vi "Teleop.vi"(10 "Match Info":T2={"Autonomous Elapsed Seconds"=0.0, "TeleOp Elapsed Seconds"=10.261, "Disabled Elapsed Seconds"=2.601, "Visited Autonomous"=FALSE, "Visited TeleOp"=TRUE, "Visited Disabled"=TRUE, "Autonomous Settings"={"Autonomous Style"=enum."Independent", "VI Refnum"=refnum}}, 11 "Call Context":T3=enum."Execute") -> ()   [LabVIEW 2014]
doc: "This VI is called for each TeleOp packet received from the DS where the robot is not disabled. It is often used to read from the joysticks and update I/O or to update setpoints for timed control loops. It should complete and return within 20 milliseconds or it may miss DS packets."
uses:
  <vilib>/Rock Robotics/WPI/DriverStation/WPI_DriverStationDerivedRobotMode.ctl
  <vilib>/Rock Robotics/WPI/DriverStation/WPI_DriverStationMatch Info.ctl
  <vilib>/Rock Robotics/WPI/RobotDrive/WPI_RobotDriveGetSetRefNum.vi
  <vilib>/Rock Robotics/WPI/Joystick/WPI_JoystickGetSetRefNum.vi
  <vilib>/Rock Robotics/Network Tables/SD Write Boolean Array.vi
  <vilib>/Rock Robotics/Network Tables/SD Write Numeric Array.vi
  <vilib>/Rock Robotics/Network Tables/SD Read Boolean.vi
  <vilib>/Rock Robotics/Network Tables/SD Read Number.vi
  <vilib>/Rock Robotics/Network Tables/SD Write Number.vi
  <vilib>/addons/control/pid/pid.llb/PID (DBL).vi
  Robot Global Data.vi
  <vilib>/addons/control/pid/NI_PID_pid.lvlib
panel:
  out "Elevator Rotation Sensor Working":bool
  out "MagneticFieldStrength2 3":u16
  out "MagneticFieldStrength2 2":u16
  out "Diag need to":u8
  out "MagnetFieldStregth":u8
  out "Rotation Sensor Data Out":u8[](array[numeric])
  out "Elevator Power":dbl
  in  "output range":cluster{"output high":dbl, "output low":dbl}={"output high"=0.7, "output low"=-0.7} {"output low" format="%.2f"; "output high" format="%.2f"}
  in  "PID gains":T1={"proportional gain (Kc)"=0.002, "integral time (Ti, min)"=0.0, "derivative time (Td, min)"=0.0} {"derivative time (Td, min)" format="%.3f"; "integral time (Ti, min)" format="%.3f"; "proportional gain (Kc)" format="%.3f"}
  in  "Move Elevator Above Tote Slide":dbl
  out "Claw Encoder Ticks":dbl
  out "Elevator Current":dbl
  out "Claw Current":dbl
  in  "Gain (VoltsPerDegree/Second)":dbl=0.0066
  in  "Reset Zero Position":bool
  out "Angle 3":dbl(knob) scale=0.0..360.0
  out "Angle 2":dbl=-0.0202788065172
  out "Angular Rate 2":dbl=-0.004938670061383929
  out "all currents (A)":dbl[](array[numeric])
  out "Elevator  Encoder Ticks":dbl
  out "Left Encoder Ticks":dbl
  out "Sample Slider 0":dbl(slide) scale=0.0..5.0
  out "Sample Boolean 1":bool
  out "Sample Boolean 0":bool
  # "Right Front"
  # "Right Rear"
  # "Elevator"
  # "Claw"
  # "Right Rear"
  # "Elevator 2"
  # "Left Front"
  # "Left Rear"
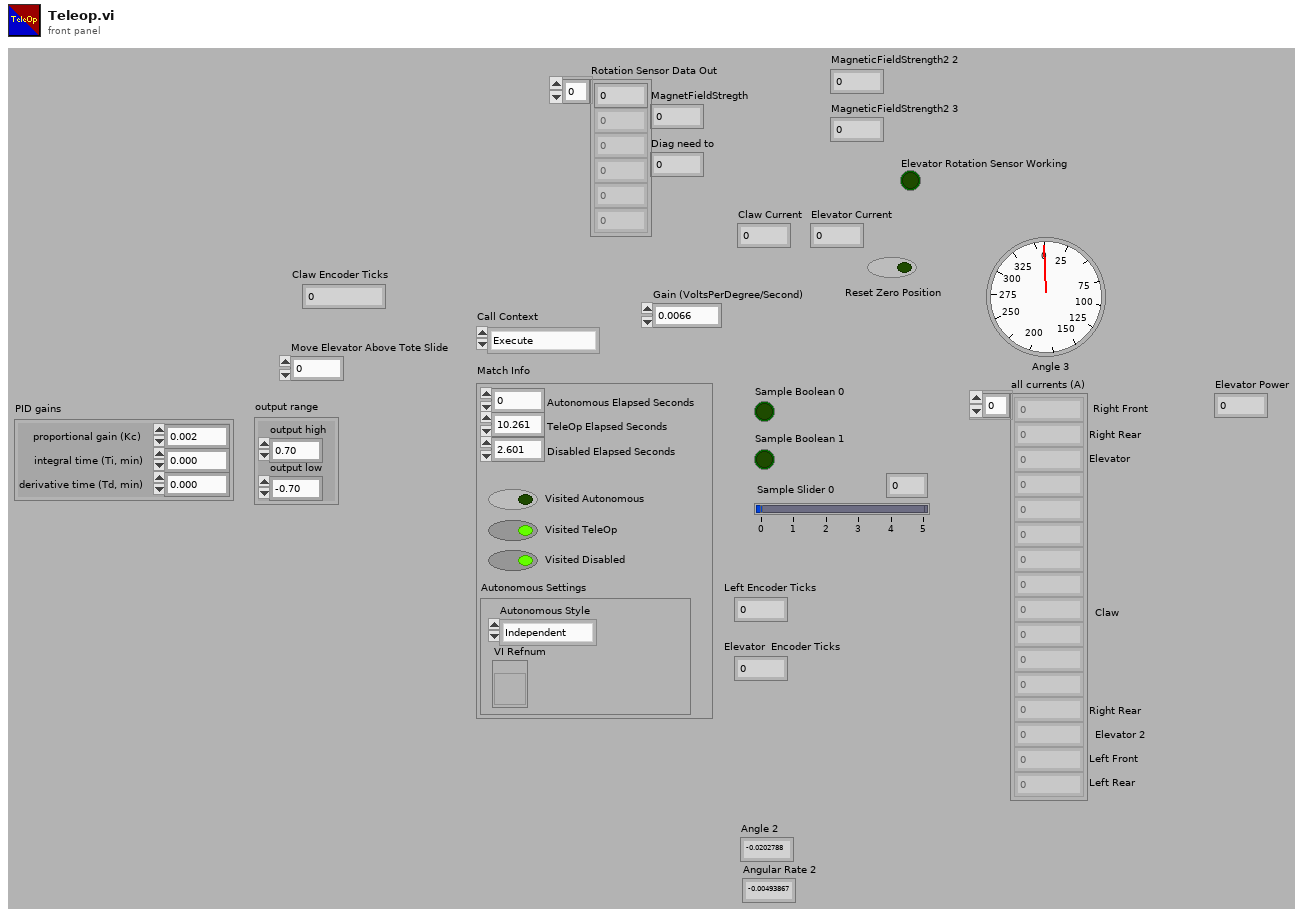
[diagram p1: front panel]
types:
  T1 = cluster{"proportional gain (Kc)":dbl, "integral time (Ti, min)":dbl, "derivative time (Td, min)":dbl}
  T2 = typedef "WPI_DriverStationMatch Info.ctl" = cluster{"Autonomous Elapsed Seconds":dbl, "TeleOp Elapsed Seconds":dbl, "Disabled Elapsed Seconds":dbl, "Visited Autonomous":bool, "Visited TeleOp":bool, "Visited Disabled":bool, "Autonomous Settings":cluster{"Autonomous Style":enum16{"Iterative", "Independent"}, "VI Refnum":refnum<vi>}}
  T3 = typedef "WPI_DriverStationDerivedRobotMode.ctl" = enum16{"Init", "Execute", "Stop"}
  T4 = typedef "WPI_RobotDriveDevRef.ctl" = cluster{"DevStatus":errorcluster, "Motors[]":T5[], "Square Inputs":bool, "Max Output":dbl}
  T5 = typedef "WPI_MotorControlDeviceRef.ctl" = cluster{"DeviceStatus":errorcluster, "Type":T6, "PWM":cluster{"Controller":T7, "PWM Channel":T8, "DeadBand":T9}, "CAN":cluster{"Device Number":u8, "Control Mode":T10, "Semaphore":T11, "Max Vout":dbl, "TalonSRX Control Mode":T12}, "Invert":bool, "TransformRef":T13, "InvTransformRef":T13}
  T6 = typedef "WPI_MotorControlType.ctl" = enum16{"PWM", "CAN", "CANTalonSRX"}
  T7 = typedef "FPGA_TypedefDigitalModule.ctl" = enum16{"Controller 1"}
  T8 = typedef "FPGA_DIOPWMChannel.ctl" = enum8{"PWM 0", "PWM 1", "PWM 2", "PWM 3", "PWM 4", "PWM 5", "PWM 6", "PWM 7", "PWM 8", "PWM 9", "PWM MXP 0", "PWM MXP 1", "PWM MXP 2", "PWM MXP 3", "PWM MXP 4", "PWM MXP 5", "PWM MXP 6", "PWM MXP 7", "PWM MXP 8", "PWM MXP 9", "Invalid"}
  T9 = typedef "WPI_PWMDeadband.ctl" = cluster{"Name":string, "maxPositivePwm":i32, "minPositivePwm":i32, "centerPwm":i32, "maxNegativePwm":i32, "minNegativePwm":i32, "angularRange":u16}
  T10 = typedef "WPI_CANJaguar_ControlMode.ctl" = enum8{"Percent VBus", "Current", "Speed", "Position", "Voltage"}
  T11 = typedef "Semaphore RefNum" = refnum<k1>
  T12 = typedef "WPI_CANTalonSRX_APIControlMode.ctl" = enum8{"Percent VBus", "Speed", "Position", "Slave", "Unchanged / Invalid"}
  T13 = typedef "WPI_PWMTransform_ConPane.ctl" = refnum<vi>
  T14 = typedef "WPI_JoystickDevRef.ctl" = cluster{"Device":T15}
  T15 = typedef "WPI_JoystickDeviceEnum.ctl" = enum16{"USB 0", "USB 1", "USB 2", "USB 3", "USB 4", "USB 5"}
  T16 = typedef "WPI_GyroDevRef.ctl" = cluster{"DevStatus":errorcluster, "Analog Module":T17, "Analog Channel":T18, "Offset":dbl, "Gain (VoltsPerDegree/Second)":dbl}
  T17 = typedef "FPGA_TypedefAnalogModule.ctl" = enum16{"Controller 1"}
  T18 = typedef "FPGA_AIChannel.ctl" = enum8{"AI 0", "AI 1", "AI 2", "AI 3", "AI MXP 0", "AI MXP 1", "AI MXP 2", "AI MXP 3", "Invalid"}
  T19 = typedef "WPI_EncoderDevRef.ctl" = cluster{"DevStatus":errorcluster, "EncoderIndex":T20, "CounterIndex":T21, "DistancePerCount":dbl, "Decoding Type":T22}
  T20 = typedef "FPGA_EncoderIdx.ctl" = enum8{"Enc 0", "Enc 1", "Enc 2", "Enc 3", "Enc 4", "Enc 5", "Enc 6", "Enc 7", "Invalid"}
  T21 = typedef "FPGA_CounterCtrSystemIndex.ctl" = enum8{"Ctr 0", "Ctr 1", "Ctr 2", "Ctr 3", "Ctr 4", "Ctr 5", "Ctr 6", "Ctr 7", "Invalid"}
  T22 = typedef "WPI_EncoderType.ctl" = enum16{"1x", "2x", "4x"}
  T23 = enum16{"Elevator State Bottom", "Elevator State Clear a Tote", "Elevator State Carry a  RC", "Elevator do Nothing"}
  T24 = enum16{"Claw State Open", "Claw State Closed", "Claw State Do Nothing", "Squeeze Hard"}
  T25 = typedef "WPI_I2CDevRef.ctl" = cluster{"DevStatus":errorcluster, "Controller":T7, "Device Address":u8, "Handle":i32, "I2C Bus":T26}
  T26 = typedef "i2c_bus.ctl" = enum16{"I2C On-Board", "I2C MXP", "Invalid"}
  T27 = cluster{"Boolean array[0]":bool, "Boolean array[1]":bool, "Boolean array[2]":bool, "Boolean array[3]":bool, "Boolean array[4]":bool, "Boolean array[5]":bool, "Boolean array[6]":bool, "Boolean array[7]":bool}
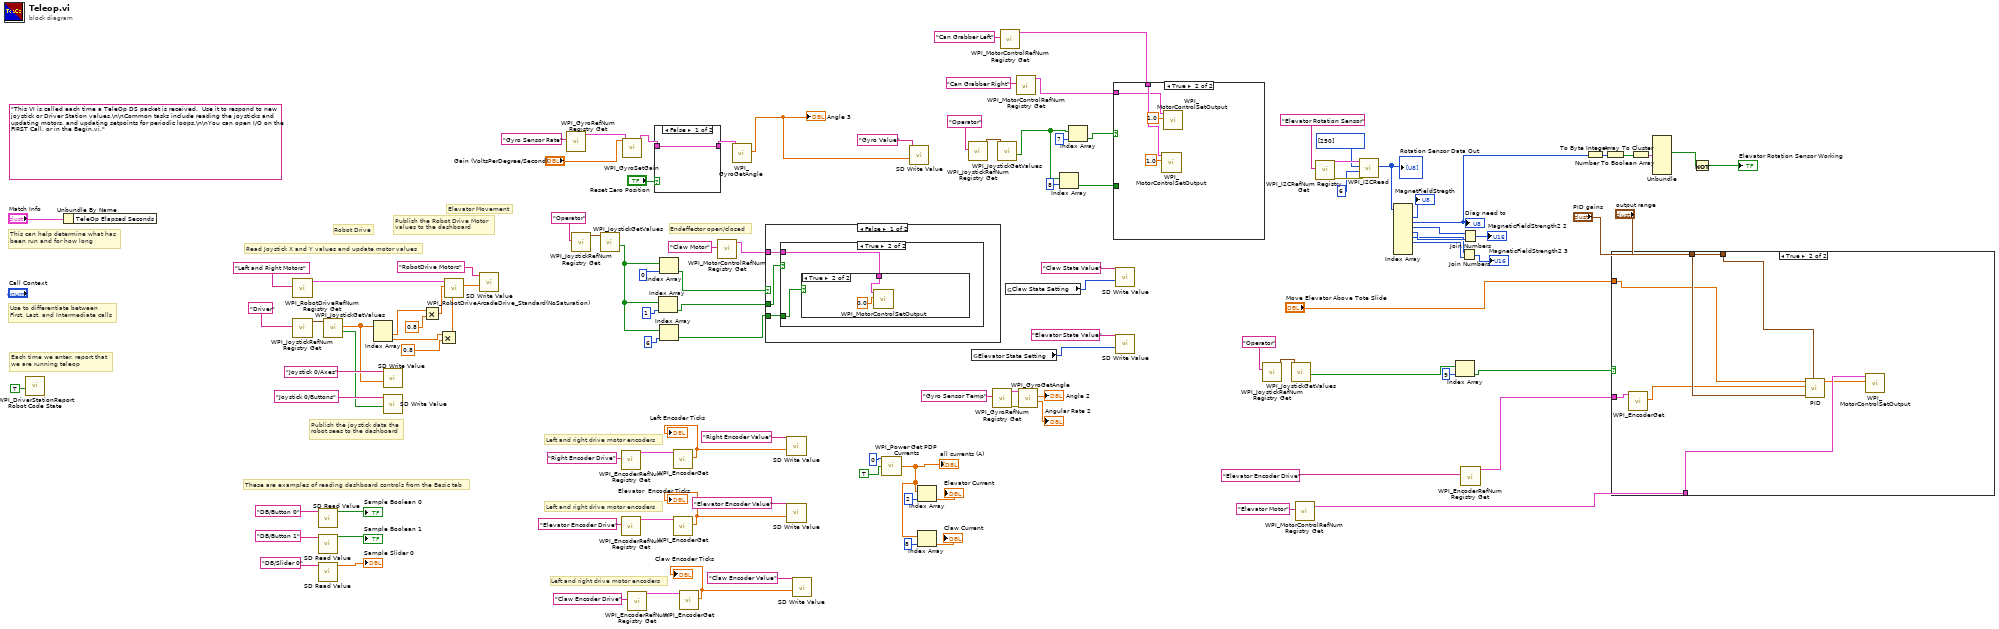
[diagram p0: block diagram]
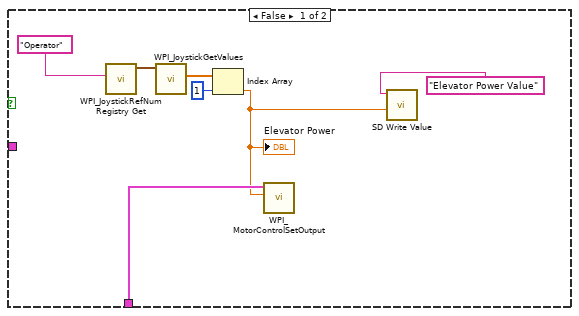
[diagram p2: hidden frame]
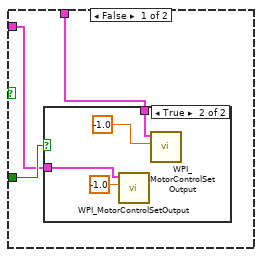
[diagram p3: hidden frame]
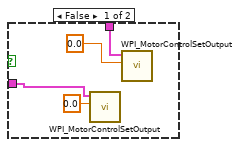
[diagram p4: hidden frame]
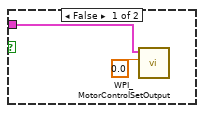
[diagram p5: hidden frame]
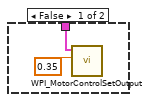
[diagram p6: hidden frame]
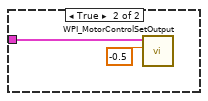
[diagram p7: hidden frame]
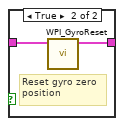
[diagram p8: hidden frame]
diagram:
  (unwired) "This VI is called each time a TeleOp DS packet is received.  Use it to respond to new joystick or Driver Station values.\n\nCommon tasks include reading the joysticks and updating motors, and updating setpoints for periodic loops.\n\nYou can open I/O on the FIRST Call, or in the Begin.vi."
  # "Left and right drive motor encoders"
  # "Endeffector open/closed"
  # "Left and right drive motor encoders"
  # "Left and right drive motor encoders"
  # "Robot Drive"
  # "Elevator Movement"
  # "These are examples of reading dashboard controls from the Basic tab"
  # "Publish the Robot Drive Motor\nvalues to the dashboard"
  # "Publish the joystick data the\nrobot sees to the dashboard"
  # "Each time we enter, report that\nwe are running teleop"
  # "Use to differentiate between\nFirst, Last, and Intermediate calls"
  # "This can help determine what has\nbeen run and for how long"
  # "Read Joystick X and Y values and update motor values"
  n1 = call <vilib>:"WPI_DriverStationReport Robot Code State.vi"("TeleOp"=TRUE ("Autonomous")) -> ()  [unwired: 10 in, 1 out]
  n2 = Unbundle By Name("Match Info") -> ()  [unwired: 1 out]
  n3 = call <vilib>:"WPI_RobotDriveRefNum Registry Get.vi"("refnum name"="Left and Right Motors") -> ("RobotDriveDevRef"=w111:T4)  [unwired: 1 in, 9 out]
  n4 = call <vilib>:"WPI_JoystickRefNum Registry Get.vi"("refnum name"="Driver") -> ("JoystickDevRef"=w109:T14)  [unwired: 1 in, 9 out]
  n5 = call-poly <vilib>:"SD Read Value.vi"("Name"="DB/Button 0" ("refnum name")) -> ("Boolean"=→"Sample Boolean 0":bool)  [unwired: 8 in, 2 out]
  n6 = call-poly <vilib>:"SD Read Value.vi"("Name"="DB/Button 1" ("refnum name")) -> ("Boolean"=→"Sample Boolean 1":bool)  [unwired: 8 in, 2 out]
  n7 = call-poly <vilib>:"SD Read Value.vi"("Name"="DB/Slider 0" ("refnum name")) -> ("Numeric"=→"Sample Slider 0":dbl)  [unwired: 8 in, 2 out]
  n8 = call <vilib>:"WPI_JoystickGetValues.vi"("JoystickDevRef"=w109) -> ("Buttons"=w96:bool[], "Axes"=w98:dbl[])  [unwired: 6 in, 3 out]
  n9 = Index Array(array=w98) -> (element #1=w88:dbl, element #2=w91:dbl)  [unwired: 2 in]
  n10 = call-poly <vilib>:"SD Write Value.vi"("Numeric Array"=w98, "Name"="Joystick 0/Axes") -> ()  [unwired: 8 in, 2 out]
  n11 = call-poly <vilib>:"SD Write Value.vi"("Boolean Array"=w96, "Name"="Joystick 0/Buttons") -> ()  [unwired: 8 in, 2 out]
  n12 = Multiply(x=w88, y=0.8) -> (x*y=w90:dbl)
  n13 = Multiply(x=w91, y=0.8) -> (x*y=w93:dbl)
  n14 = call <vilib>:"WPI_RobotDriveArcadeDrive_Standard(NoSaturation).vi"("Y axis value"=w93, "X axis value"=w90, "RobotDriveDevRef"=w111) -> ("Motor Values"=w100:dbl[])  [unwired: 1 in, 7 out]
  n15 = call-poly <vilib>:"SD Write Value.vi"("Numeric Array"=w100, "Name"="RobotDrive Motors") -> ()  [unwired: 8 in, 2 out]
  n16 = call <vilib>:"WPI_GyroRefNum Registry Get.vi"("refnum name"="Gyro Sensor Rate") -> ("GyroDevRef"=w70:T16)  [unwired: 9 in, 1 out]
  n17 = call <vilib>:"WPI_JoystickRefNum Registry Get.vi"("refnum name"="Operator") -> ("JoystickDevRef"=w69:T14)  [unwired: 1 in, 9 out]
  n18 = call <vilib>:"WPI_JoystickGetValues.vi"("JoystickDevRef"=w69) -> ("Buttons"=w46:bool[])  [unwired: 6 in, 4 out]
  n19 = call <vilib>:"WPI_EncoderRefNum Registry Get.vi"("refnum name"="Right Encoder Drive") -> ("EncoderDevRef"=w94:T19)  [unwired: 9 in, 1 out]
  n20 = call <vilib>:"WPI_EncoderRefNum Registry Get.vi"("refnum name"="Elevator Encoder Drive") -> ("EncoderDevRef"=w83:T19)  [unwired: 9 in, 1 out]
  n21 = call <vilib>:"WPI_GyroSetGain.vi"("Gain (VoltsPerDegree/Second)"="Gain (VoltsPerDegree/Second)", "GyroDevRef"=w70) -> ("GyroDevRef"=w74:T16)  [unwired: 1 in, 8 out]
  n22 = call <vilib>:"WPI_EncoderRefNum Registry Get.vi"("refnum name"="Claw Encoder Drive") -> ("EncoderDevRef"=w49:T19)  [unwired: 9 in, 1 out]
  n23 = case shown="False" "Reset Zero Position" {
    tunnel: w74 -> [w114 w116]
    tunnel: [w114 w115] -> w71
    frame False {
    }
    frame True {
      # "Reset gyro zero \nposition"
      n24 = call <vilib>:"WPI_GyroReset.vi"("GyroDevRef"=w116) -> ("GyroDevRef"=w115:T16)  [unwired: 10 out]
    }
  }
  n25 = Index Array(array=w46, index=1) -> (element=w64:bool)
  n26 = Index Array(array=w46, index=0) -> (element=w65:bool)
  n27 = Index Array(array=w46, index=6) -> (element=w45:bool)
  n28 = call <vilib>:"WPI_EncoderGet.vi"("EncoderDevRef"=w94) -> ("Distance"=w86:dbl)  [unwired: 5 in, 5 out]
  "Left Encoder Ticks" <- w86
  n29 = call <vilib>:"WPI_EncoderGet.vi"("EncoderDevRef"=w83) -> ("Distance"=w85:dbl)  [unwired: 5 in, 5 out]
  "Elevator  Encoder Ticks" <- w85
  n30 = call <vilib>:"WPI_EncoderGet.vi"("EncoderDevRef"=w49) -> ("Distance"=w51:dbl)  [unwired: 5 in, 5 out]
  "Claw Encoder Ticks" <- w51
  n31 = call <vilib>:"WPI_MotorControlRefNum Registry Get.vi"("refnum name"="Claw Motor") -> ("MotorControlDevRef"=w44:T5)  [unwired: 9 in, 1 out]
  n32 = call <vilib>:"WPI_GyroGetAngle.vi"("GyroDevRef"=w71) -> ("Angle"=w52:dbl)  [unwired: 1 in, 9 out]
  "Angle 3" <- w52
  n33 = case shown="False" w65 {
    tunnel: w64 -> [w119 _]
    tunnel: w45 -> [w118 _]
    tunnel: w44 -> [w117 w129]
    frame False {
      n34 = case shown="True" w119 {
        tunnel: w118 -> [_ w123]
        tunnel: w117 -> [w120 w122]
        frame False {
          n35 = call <vilib>:"WPI_MotorControlSetOutput.vi"("Output"=0.0, "MotorControlDevRef"=w120) -> ()  [unwired: 7 in, 3 out]
        }
        frame True {
          n36 = case shown="True" w123 {
            tunnel: w122 -> [w124 w127]
            frame False {
              n37 = call <vilib>:"WPI_MotorControlSetOutput.vi"("Output"=0.35, "MotorControlDevRef"=w124) -> ()  [unwired: 7 in, 3 out]
            }
            frame True {
              n38 = call <vilib>:"WPI_MotorControlSetOutput.vi"("Output"=0.0, "MotorControlDevRef"=w127) -> ()  [unwired: 7 in, 3 out]
            }
          }
        }
      }
    }
    frame True {
      n39 = call <vilib>:"WPI_MotorControlSetOutput.vi"("Output"=-0.5, "MotorControlDevRef"=w129) -> ()  [unwired: 7 in, 3 out]
    }
  }
  n40 = call-poly <vilib>:"SD Write Value.vi"("Numeric"=w86, "Name"="Right Encoder Value") -> ()  [unwired: 8 in, 2 out]
  n41 = call-poly <vilib>:"SD Write Value.vi"("Numeric"=w85, "Name"="Elevator Encoder Value") -> ()  [unwired: 8 in, 2 out]
  n42 = call-poly <vilib>:"SD Write Value.vi"("Numeric"=w51, "Name"="Claw Encoder Value") -> ()  [unwired: 8 in, 2 out]
  n43 = call <vilib>:"WPI_Power Get PDP Currents.vi"("Power Distribution Panel (0)"=u8 0, "Tare Currents?"=TRUE) -> ("all currents (A)"=w62:dbl[])  [unwired: 11 in, 2 out]
  "all currents (A)" <- w62
  n44 = call-poly <vilib>:"SD Write Value.vi"("Numeric"=w52, "Name"="Gyro Value") -> ()  [unwired: 8 in, 2 out]
  n45 = Index Array(array=w62, index=8) -> (element=→"Claw Current":dbl)
  n46 = Index Array(array=w62, index=2) -> (element=→"Elevator Current":dbl)
  n47 = call <vilib>:"WPI_JoystickRefNum Registry Get.vi"("refnum name"="Operator") -> ("JoystickDevRef"=w40:T14)  [unwired: 1 in, 9 out]
  n48 = global read "Robot Global Data.vi" "Elevator State Setting"() -> (w55:T23)
  n49 = call <vilib>:"WPI_GyroRefNum Registry Get.vi"("refnum name"="Gyro Sensor Temp") -> ("error out"=w76:errorcluster, "GyroDevRef"=w77:T16)  [unwired: 9 in]
  n50 = call <vilib>:"WPI_JoystickGetValues.vi"("JoystickDevRef"=w40) -> ("Buttons"=w32:bool[])  [unwired: 6 in, 4 out]
  n51 = call <vilib>:"WPI_MotorControlRefNum Registry Get.vi"("refnum name"="Can Grabber Left") -> ("MotorControlDevRef"=w35:T5)  [unwired: 9 in, 1 out]
  n52 = global read "Robot Global Data.vi" "Claw State Setting"() -> (w56:T24)
  n53 = call <vilib>:"WPI_MotorControlRefNum Registry Get.vi"("refnum name"="Can Grabber Right") -> ("MotorControlDevRef"=w38:T5)  [unwired: 9 in, 1 out]
  n54 = call <vilib>:"WPI_GyroGetAngle.vi"("error in (no error)"=w76, "GyroDevRef"=w77) -> ("Angular Rate"=→"Angular Rate 2":dbl, "Angle"=→"Angle 2":dbl)  [unwired: 6 in, 2 out]
  n55 = Index Array(array=w32, index=8) -> (element=w33:bool)
  n56 = Index Array(array=w32, index=7) -> (element=w42:bool)
  n57 = case shown="True" w42 {
    tunnel: w38 -> [w131 w141]
    tunnel: w35 -> [w130 w142]
    tunnel: w33 -> [w132 _]
    frame False {
      n58 = case shown="True" w132 {
        tunnel: w131 -> [w134 w138]
        tunnel: w130 -> [w133 w137]
        frame False {
          n59 = call <vilib>:"WPI_MotorControlSetOutput.vi"("Output"=0.0, "MotorControlDevRef"=w134) -> ()  [unwired: 7 in, 3 out]
          n60 = call <vilib>:"WPI_MotorControlSetOutput.vi"("Output"=0.0, "MotorControlDevRef"=w133) -> ()  [unwired: 7 in, 3 out]
        }
        frame True {
          n61 = call <vilib>:"WPI_MotorControlSetOutput.vi"("Output"=-1.0, "MotorControlDevRef"=w138) -> ()  [unwired: 7 in, 3 out]
          n62 = call <vilib>:"WPI_MotorControlSetOutput.vi"("Output"=-1.0, "MotorControlDevRef"=w137) -> ()  [unwired: 7 in, 3 out]
        }
      }
    }
    frame True {
      n63 = call <vilib>:"WPI_MotorControlSetOutput.vi"("Output"=1.0, "MotorControlDevRef"=w142) -> ()  [unwired: 7 in, 3 out]
      n64 = call <vilib>:"WPI_MotorControlSetOutput.vi"("Output"=1.0, "MotorControlDevRef"=w141) -> ()  [unwired: 7 in, 3 out]
    }
  }
  n65 = call-poly <vilib>:"SD Write Value.vi"("Numeric"=w56, "Name"="Claw State Value") -> ()  [unwired: 8 in, 2 out]
  n66 = call-poly <vilib>:"SD Write Value.vi"("Numeric"=w55, "Name"="Elevator State Value") -> ()  [unwired: 8 in, 2 out]
  n67 = call <vilib>:"WPI_JoystickRefNum Registry Get.vi"("refnum name"="Operator") -> ("JoystickDevRef"=w24:T14)  [unwired: 1 in, 9 out]
  n68 = call <vilib>:"WPI_JoystickGetValues.vi"("JoystickDevRef"=w24) -> ("Buttons"=w22:bool[])  [unwired: 6 in, 4 out]
  n69 = call <vilib>:"WPI_MotorControlRefNum Registry Get.vi"("refnum name"="Elevator Motor") -> ("MotorControlDevRef"=w27:T5)  [unwired: 9 in, 1 out]
  n70 = call <vilib>:"WPI_I2CRefNum Registry Get.vi"("refnum name"="Elevator Rotation Sensor") -> ("error out"=w17:errorcluster, "I2CDevRef"=w19:T25)  [unwired: 9 in]
  n71 = call <vilib>:"WPI_I2CRead.vi"("error in (no error)"=w17, "I2CBytesToRead"=u8 6, "I2CRegister"=u8[] [250], "I2CDevRef"=w19) -> ("Data Out"=w14:u8[])  [unwired: 5 in, 2 out]
  "Rotation Sensor Data Out" <- w14
  n72 = Index Array(array=w14) -> (element #1=→"MagnetFieldStregth":u8, element #2=w4:u8, element #3=w11:u8, element #4=w10:u8, element #5=w9:u8, element #6=w8:u8)  [unwired: 8 in, 2 out]
  "Diag need to" <- w4
  n73 = Index Array(array=w22, index=9) -> (element=w20:bool)
  n74 = Join Numbers(hi=w9, lo=w8) -> ((hi.lo)=→"MagneticFieldStrength2 3":u16)
  n75 = Join Numbers(hi=w11, lo=w10) -> ((hi.lo)=→"MagneticFieldStrength2 2":u16)
  n76 = call <vilib>:"WPI_EncoderRefNum Registry Get.vi"("refnum name"="Elevator Encoder Drive") -> ("EncoderDevRef"=w25:T19)  [unwired: 9 in, 1 out]
  n77 = To Byte Integer(number=w4) -> (8bit integer=w5:i8)
  n78 = Number To Boolean Array(number=w5) -> (Boolean array=w3:bool[])
  n79 = case shown="True" w20 {
    tunnel: "output range" -> [_ w154]
    tunnel: "PID gains" -> [_ w158]
    tunnel: w25 -> [_ w157]
    tunnel: w27 -> [w146 w155]
    tunnel: "Move Elevator Above Tote Slide" -> [_ w153]
    frame False {
      n80 = call <vilib>:"WPI_JoystickRefNum Registry Get.vi"("refnum name"="Operator") -> ("JoystickDevRef"=w151:T14)  [unwired: 1 in, 9 out]
      n81 = call <vilib>:"WPI_JoystickGetValues.vi"("JoystickDevRef"=w151) -> ("Axes"=w149:dbl[])  [unwired: 6 in, 4 out]
      n82 = Index Array(array=w149, index=1) -> (element=w145:dbl)
      "Elevator Power" <- w145
      n83 = call <vilib>:"WPI_MotorControlSetOutput.vi"("Output"=w145, "MotorControlDevRef"=w146) -> ()  [unwired: 7 in, 3 out]
      n84 = call-poly <vilib>:"SD Write Value.vi"("Numeric"=w145, "Name"="Elevator Power Value") -> ()  [unwired: 8 in, 2 out]
    }
    frame True {
      n85 = call <vilib>:"WPI_EncoderGet.vi"("EncoderDevRef"=w157) -> ("Distance"=w156:dbl)  [unwired: 5 in, 5 out]
      n86 = call-poly <vilib>:"PID.vi"("output range"=w154, "PID gains"=w158, "process variable"=w156, "setpoint"=w153) -> ("output"=w152:dbl)  [unwired: 6 in, 1 out]
      n87 = call <vilib>:"WPI_MotorControlSetOutput.vi"("Output"=w152, "MotorControlDevRef"=w155) -> ()  [unwired: 7 in, 3 out]
    }
  }
  n88 = Array To Cluster(array=w3) -> (cluster=w6:T27)
  n89 = Unbundle(w6) -> ("Boolean array[3]"=w2:bool)  [unwired: 7 out]
  n90 = Not(x=w2) -> (.not. x?=→"Elevator Rotation Sensor Working":bool)
